vi "HotLotDataToExcel.vi"(9 "Header":string, 11 "data":string[][](array[string])) -> ()   [LabVIEW 2012]
uses:
  <vilib>/Utility/NIReport.llb/NI_report.lvclass
  Global1.vi
  <vilib>/Utility/NIReport.llb/Excel/NI_Excel.lvclass
panel:
  out "error out 4":errorcluster
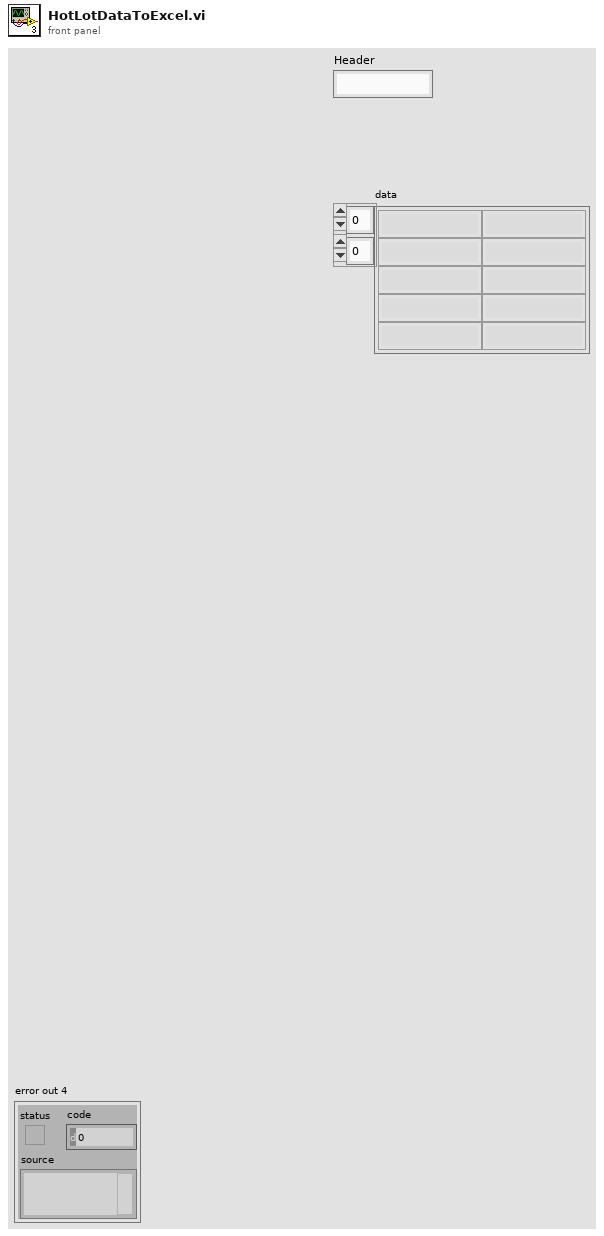
[diagram p1: front panel]
types:
  T1 = enum16{"Standard Report", "HTML", "Word", "Excel"}
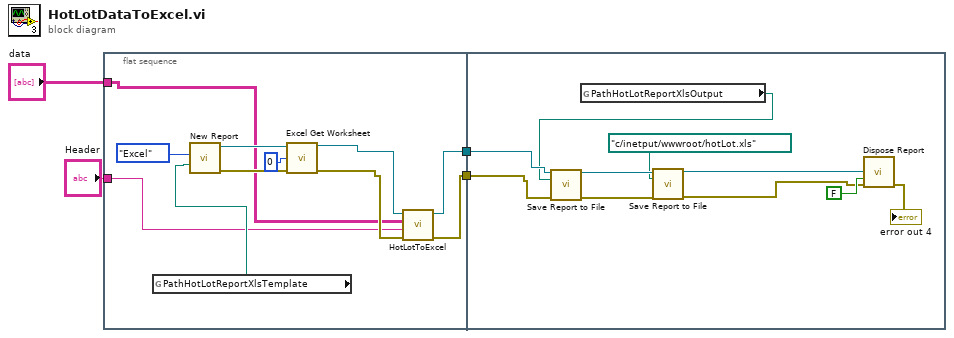
[diagram p0: block diagram]
diagram:
  n1 = flat-sequence {
    tunnel: "Header" -> [w6]
    tunnel: [w8] -> w4
    tunnel: [w7] -> w3
    tunnel: "data" -> [w5]
    tunnel: w4 -> [w23]
    tunnel: w3 -> [w22]
    frame #0 {
      n2 = global read "Global1.vi" "PathHotLotReportXlsTemplate"() -> (w11:path)
      n3 = call <vilib>:"New Report.vi"("report type"=T1."Excel" ("Report Type"), "template (empty)"=w11) -> ("report out"=w14:refnum<class "NI_report.lvclass">, "error out"=w13:errorcluster)  [unwired: 12 in]
      n4 = call <vilib>:"Excel Get Worksheet.vi"("report in"=w14, "worksheet index (0)"=0, "error in (no error)"=w13) -> ("report out"=w10:refnum<class "NI_report.lvclass">, "error out"=w9:errorcluster)  [unwired: 11 in]
      n5 = call "HotLotToExcel.vi"("error in (no error)"=w9, "Header"=w6, "Input"=w5, "report in"=w10) -> ("error out"=w7:errorcluster, "report out"=w8:refnum<class "NI_report.lvclass">)  [unwired: 6 in]
    }
    frame #1 {
      n6 = global read "Global1.vi" "PathHotLotReportXlsOutput"() -> (w21:path)
      n7 = call-dynamic "Save Report to File.vi"("report in"=w23, "report file path"=w21, "error in (no error)"=w22) -> ("report out"=w20:refnum<class "NI_report.lvclass">, "error out"=w18:errorcluster)  [unwired: 11 in]
      n8 = call-dynamic "Save Report to File.vi"("report in"=w20, "report file path"=path "c:/inetput/wwwroot/hotLot.xls", "error in (no error)"=w18) -> ("report out"=w19:refnum<class "NI_report.lvclass">, "error out"=w17:errorcluster)  [unwired: 11 in]
      n9 = call-dynamic "Dispose Report.vi"("report in"=w19, "save changes? (F)"=FALSE, "error in (no error)"=w17) -> ("error out"=→"error out 4":errorcluster)  [unwired: 12 in]
    }
  }
